vi "DELETETest.vi"() -> ()   [LabVIEW 2019]
uses:
  Instrument.DAQ/Typedefs/Results--Cluster.ctl
  Instrument.DAQ/Instrument.DAQ.lvclass
  Instrument.DAQ/Typedefs/REF.Channel--Cluster.ctl
  Instrument.DAQ/Typedefs/DAQ.Sampling.Sampling--Cluster.ctl
  Instrument.DAQ/Instrument.DAQ.lvclass/Instrument.DAQ.ctl
  C:/Program Files/National Instruments/LabVIEW 2019/vi.lib/JKI/JKI SMO/SMO/SMO.lvclass
panel:
  out "Waveform Graph 2":dbl[][](graph)
  out "Waveform Graph":waveform(dbl)[](graph)
  out "<Results> (X,Y,R,Theta,Mean)":T1 {"Results (Dictionary)"."value" format="%#_6p"}
  out "error out":errorcluster
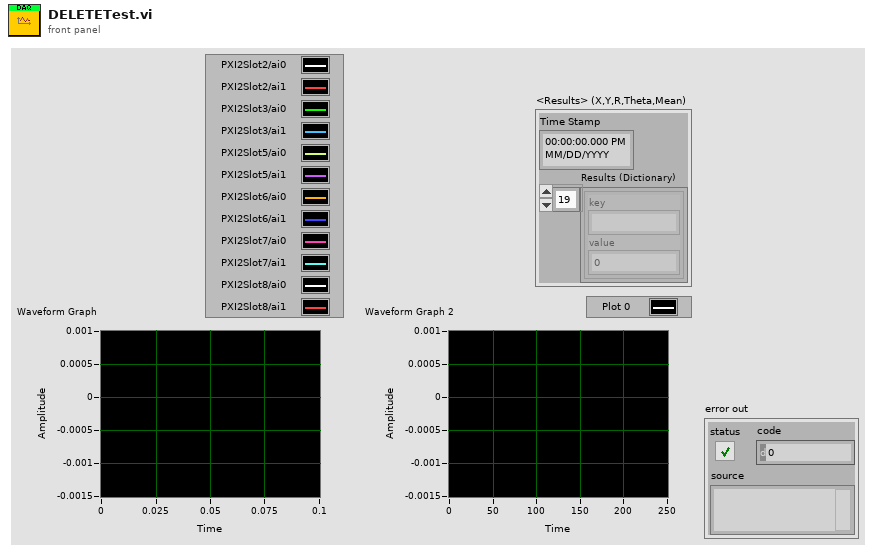
[diagram p1: front panel]
types:
  T1 = typedef "Instrument.Lockin.lvlib/Instrument.DAQ.lvclass/Results--Cluster.ctl" = cluster{"Time Stamp":timestamp, "Results (Dictionary)":cluster{"key":string, "value":dbl}[]}
  T2 = typedef "Instrument.Lockin.lvlib/Instrument.DAQ.lvclass/DAQ.Sampling.Sampling--Cluster.ctl" = cluster{"Fs":dbl, "#s":i32}
  T3 = typedef "Instrument.Lockin.lvlib/Instrument.DAQ.lvclass/REF.Channel--Cluster.ctl" = cluster{"Enable?":bool, "Channel":i32, "Frequency":dbl, "Phase":dbl, "TC":dbl, "Roll-Off":i32}
  T4 = cluster{"Enable?":bool, "Channel":i32, "References":i32[]}[]
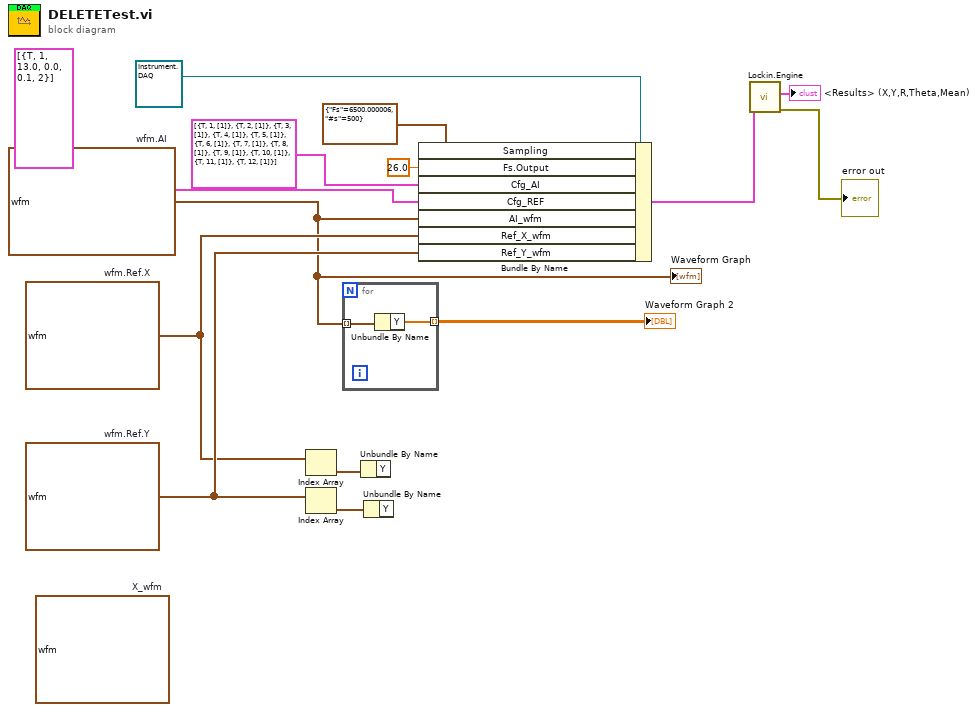
[diagram p0: block diagram]
diagram:
  (unwired) waveform(dbl)[] [{"t0"=timestamp(3836122117.000668 s since 1904-01-01), "dt"=7.692307684820775e-05, "Y"=array[1000 elements], "attributes"=variant("AI Channel"=variant(i32 1), "Quadrature"=variant(string "X"), "Reference Channel"=variant(i32 1))}, {"t0"=timestamp(3836122117.000668 s since 1904-01-01), "dt"=7.692307684820775e-05, "Y"=array[1000 elements], "attributes"=variant("AI Channel"=variant(i32 2), "Quadrature"=variant(string "X"), "Reference Channel"=variant(i32 1))}, {"t0"=timestamp(3836122117.000668 s since 1904-01-01), "dt"=7.692307684820775e-05, "Y"=array[1000 elements], "attributes"=variant("AI Channel"=variant(i32 3), "Quadrature"=variant(string "X"), "Reference Channel"=variant(i32 1))}, {"t0"=timestamp(3836122117.000668 s since 1904-01-01), "dt"=7.692307684820775e-05, "Y"=array[1000 elements], "attributes"=variant("AI Channel"=variant(i32 4), "Quadrature"=variant(string "X"), "Reference Channel"=variant(i32 1))}]  # X_wfm
  w5 = waveform(dbl)[] [{"t0"=timestamp(3755872525.694636 s since 1904-01-01), "dt"=0.000307692307392831, "Y"=array[250 elements], "attributes"=variant("Reference Channel"=variant(i32 1))}]  # wfm.Ref.X
  w6 = waveform(dbl)[] [{"t0"=timestamp(3755872531.157137 s since 1904-01-01), "dt"=0.000307692307392831, "Y"=array[250 elements], "attributes"=variant("Reference Channel"=variant(i32 1))}]  # wfm.Ref.Y
  w1 = waveform(dbl)[] [{"t0"=timestamp(3755872515.131535 s since 1904-01-01), "dt"=0.00030769230739283095, "Y"=array[250 elements], "attributes"=variant("NI_ChannelName"=variant(string "PXI2Slot2/ai0"), "NI_UnitDescription"=variant(string "Volts"))}, {"t0"=timestamp(3755872515.131535 s since 1904-01-01), "dt"=0.00030769230739283095, "Y"=array[250 elements], "attributes"=variant("NI_ChannelName"=variant(string "PXI2Slot2/ai1"), "NI_UnitDescription"=variant(string "Volts"))}, {"t0"=timestamp(3755872515.131535 s since 1904-01-01), "dt"=0.00030769230739283095, "Y"=array[250 elements], "attributes"=variant("NI_ChannelName"=variant(string "PXI2Slot3/ai0"), "NI_UnitDescription"=variant(string "Volts"))}, {"t0"=timestamp(3755872515.131535 s since 1904-01-01), "dt"=0.00030769230739283095, "Y"=array[250 elements], "attributes"=variant("NI_ChannelName"=variant(string "PXI2Slot3/ai1"), "NI_UnitDescription"=variant(string "Volts"))}, {"t0"=timestamp(3755872515.131535 s since 1904-01-01), "dt"=0.00030769230739283095, "Y"=array[250 elements], "attributes"=variant("NI_ChannelName"=variant(string "PXI2Slot5/ai0"), "NI_UnitDescription"=variant(string "Volts"))}, {"t0"=timestamp(3755872515.131535 s since 1904-01-01), "dt"=0.00030769230739283095, "Y"=array[250 elements], "attributes"=variant("NI_ChannelName"=variant(string "PXI2Slot5/ai1"), "NI_UnitDescription"=variant(string "Volts"))}, {"t0"=timestamp(3755872515.131535 s since 1904-01-01), "dt"=0.00030769230739283095, "Y"=array[250 elements], "attributes"=variant("NI_ChannelName"=variant(string "PXI2Slot6/ai0"), "NI_UnitDescription"=variant(string "Volts"))}, {"t0"=timestamp(3755872515.131535 s since 1904-01-01), "dt"=0.00030769230739283095, "Y"=array[250 elements], "attributes"=variant("NI_ChannelName"=variant(string "PXI2Slot6/ai1"), "NI_UnitDescription"=variant(string "Volts"))}, {"t0"=timestamp(3755872515.131535 s since 1904-01-01), "dt"=0.00030769230739283095, "Y"=array[250 elements], "attributes"=variant("NI_ChannelName"=variant(string "PXI2Slot7/ai0"), "NI_UnitDescription"=variant(string "Volts"))}, {"t0"=timestamp(3755872515.131535 s since 1904-01-01), "dt"=0.00030769230739283095, "Y"=array[250 elements], "attributes"=variant("NI_ChannelName"=variant(string "PXI2Slot7/ai1"), "NI_UnitDescription"=variant(string "Volts"))}, {"t0"=timestamp(3755872515.131535 s since 1904-01-01), "dt"=0.00030769230739283095, "Y"=array[250 elements], "attributes"=variant("NI_ChannelName"=variant(string "PXI2Slot8/ai0"), "NI_UnitDescription"=variant(string "Volts"))}, {"t0"=timestamp(3755872515.131535 s since 1904-01-01), "dt"=0.00030769230739283095, "Y"=array[250 elements], "attributes"=variant("NI_ChannelName"=variant(string "PXI2Slot8/ai1"), "NI_UnitDescription"=variant(string "Volts"))}]  # wfm.AI
  n1 = Index Array(array=w5) -> (element=w4:waveform(dbl))  [unwired: 1 in]
  n2 = Index Array(array=w6) -> (element=w3:waveform(dbl))  [unwired: 1 in]
  n3 = for {
    tunnel: w1 -> [w16] mode=indexing
    tunnel: [w15] -> w2 mode=indexing
    n4 = Unbundle By Name(w16) -> ("Y"=w15:dbl[])
  }
  "Waveform Graph 2" <- w2
  n5 = Unbundle By Name(w4) -> ()  [unwired: 1 out]
  n6 = Unbundle By Name(w3) -> ()  [unwired: 1 out]
  n7 = Bundle By Name(cluster=refnum<class "Instrument.DAQ.lvclass"> refnum ("Instrument.DAQ"), "Sampling"=T2 {"Fs"=6500.000006, "#s"=500} ("Configuration.DAQ.Sampling.Sampling"), "Fs.Output"=26.0 ("Configuration.DAQ.Sampling.Fs.Output"), "Cfg_AI"=T4 [{"Enable?"=TRUE, "Channel"=1, "References"=[1]}, {"Enable?"=TRUE, "Channel"=2, "References"=[1]}, {"Enable?"=TRUE, "Channel"=3, "References"=[1]}, {"Enable?"=TRUE, "Channel"=4, "References"=[1]}, {"Enable?"=TRUE, "Channel"=5, "References"=[1]}, {"Enable?"=TRUE, "Channel"=6, "References"=[1]}, {"Enable?"=TRUE, "Channel"=7, "References"=[1]}, {"Enable?"=TRUE, "Channel"=8, "References"=[1]}, {"Enable?"=TRUE, "Channel"=9, "References"=[1]}, {"Enable?"=TRUE, "Channel"=10, "References"=[1]}, {"Enable?"=TRUE, "Channel"=11, "References"=[1]}, {"Enable?"=TRUE, "Channel"=12, "References"=[1]}] ("Cfg.AI"), "Cfg_REF"=T3[] [{"Enable?"=TRUE, "Channel"=1, "Frequency"=13.0, "Phase"=0.0, "TC"=0.1, "Roll-Off"=2}], "AI_wfm"=w1, "Ref_X_wfm"=w5, "Ref_Y_wfm"=w6) -> (w13:cluster{})
  n8 = call "Lockin.Engine.vi"("Instrument.DAQ"=w13) -> ("error out"=→"error out":errorcluster, "<Results> (X,Y,R,Theta,Mean)"=→"<Results> (X,Y,R,Theta,Mean)":T1)  [unwired: 8 in, 1 out]
  "Waveform Graph" <- w1
